vi "Power-On Status Query.vi"(0 "VISA resource name":refnum<visa-resource-name>, 11 "error in (no error)":errorcluster) -> (4 "VISA resource name out":refnum<visa-resource-name>, 6 "Power On Status":u16(ring) items=["Power-On Load Previous Enable Registers", "Power-On Clear Enable Registers"], 15 "error out":errorcluster)   [LabVIEW 2020, in "eec 6700.lvlib"]
doc: "Queries the power-on status clear setting. Returns 0 or 1"
uses:
  <instrlib>/eec 6700/eec 6700.lvlib
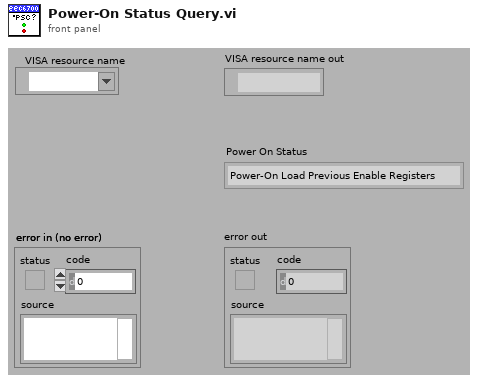
[diagram p1: front panel]
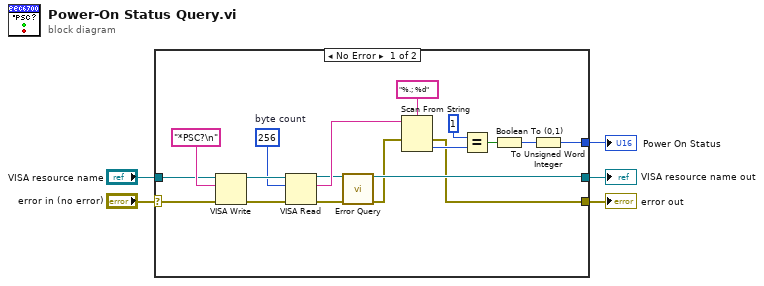
[diagram p0: block diagram]
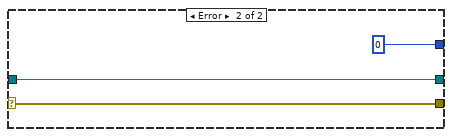
[diagram p2: hidden frame]
diagram:
  n1 = case shown="No Error" "error in (no error)" {
    selector: "error in (no error)" -> [w12 w25]
    tunnel: [w11 i16 0] -> w5
    tunnel: "VISA resource name" -> [w14 w26]
    tunnel: [w10 w26] -> w3
    tunnel: [w7 w25] -> w2
    frame No Error {
      w16 = u32 256  # byte count
      n2 = VISA Write(VISA resource name=w14, write buffer="*PSC?\n" ("Command to Send (empty)"), error in (no error)=w12) -> (VISA resource name out=w18:refnum<visa-resource-name>, error out=w17:errorcluster)  [unwired: 1 out]
      n3 = VISA Read(VISA resource name=w18, byte count=w16, error in (no error)=w17) -> (VISA resource name out=w9:refnum<visa-resource-name>, read buffer=w13:string, error out=w6:errorcluster)  [unwired: 1 out]
      n4 = call <instrlib>:"Error Query.vi"("VISA resource name"=w9, "error in (no error)"=w6) -> ("VISA resource name out"=w10:refnum<visa-resource-name>, "error out"=w8:errorcluster)  [unwired: 10 in, 2 out]
      n5 = Scan From String(format string="%.; %d" ("Format String"), input string=w13, error in=w8) -> (error out=w7:errorcluster, output 1=w22:i32)  [unwired: 2 in, 2 out]
      n6 = Equal?(x=1, y=w22) -> (x = y?=w20:bool)
      n7 = Boolean To (0,1)(Boolean=w20) -> (0, 1=w19:i16)
      n8 = To Unsigned Word Integer(number=w19) -> (unsigned 16bit integer=w11:u16)
    }
    frame Error {
    }
  }
  "Power On Status" <- w5
  "VISA resource name out" <- w3
  "error out" <- w2
